vi "Continuous Distillation.vi"() -> ()   [LabVIEW 2017]
uses:
  Halt ContD.vi
  <vilib>/addons/control/pid/pid.llb/PID Advanced (DBL).vi
  <vilib>/addons/control/pid/NI_PID_pid.lvlib
panel:
  out "Condenser Pressure":dbl caption="mbar" format="%#.0f"
  out "Feed Tank Weight":dbl caption="Kg" format="%#.2f"
  in  "Bottoms Flowrate":dbl caption="%"
  in  "Td (Feed Temp)":dbl caption="(min)" format="%.2g"
  in  "Ti (Feed Temp)":dbl=7.0 caption="(min)" format="%.2g"
  in  "Kc (Feed Temp)":dbl=2.0 format="%.2g"
  in  "Reflux Flowrate":dbl caption="ml/min" format="%.1g"
  in  "Feed Flowrate":dbl caption="ml/min" format="%.1g"
  in  "Main Power":bool
  in  "Set Manual Feed Preheater Output":dbl(slide) scale=0.0..100.0
  in  "Manual Control Override":bool
  out "Feed Preheater Output":dbl(slide)=17.346938775510203 scale=0.0..100.0
  in  "Feed Temperature Setpoint":dbl caption="C" format="%.1f"
  out "Feed Temperature":dbl format="%.1g"
  in  "Reboiler Duty":dbl caption="watts"
  out "Tray 11 Temperature":dbl format="%.1g"
  out "Reboiler Temperature":dbl format="%.1g"
  out "Reflux Temperature":dbl format="%.1g"
  out "Overhead Vapor Temperature":dbl caption="C" format="%.1f"
  out "Tray 4 Temperature":dbl caption="C" format="%.1f"
  out "Reboiler Pressure":dbl caption="mbar"
  out "Approximate Bottoms Composition":dbl caption="Wt% CH3OH" format="%.1f"
  out "Approximate Distillate Composition":dbl caption="Wt% CH3OH" format="%.1f"
  in  "stop":bool
  out "Data Point Count":i32
  in  "Specify Time between Data Points (sec)":dbl=1.0
  in  "Cancel Data Collection":bool
  in  "Specify number of data points":i16=1
  in  "Enable 3":bool
  out "Saving Data 3":bool
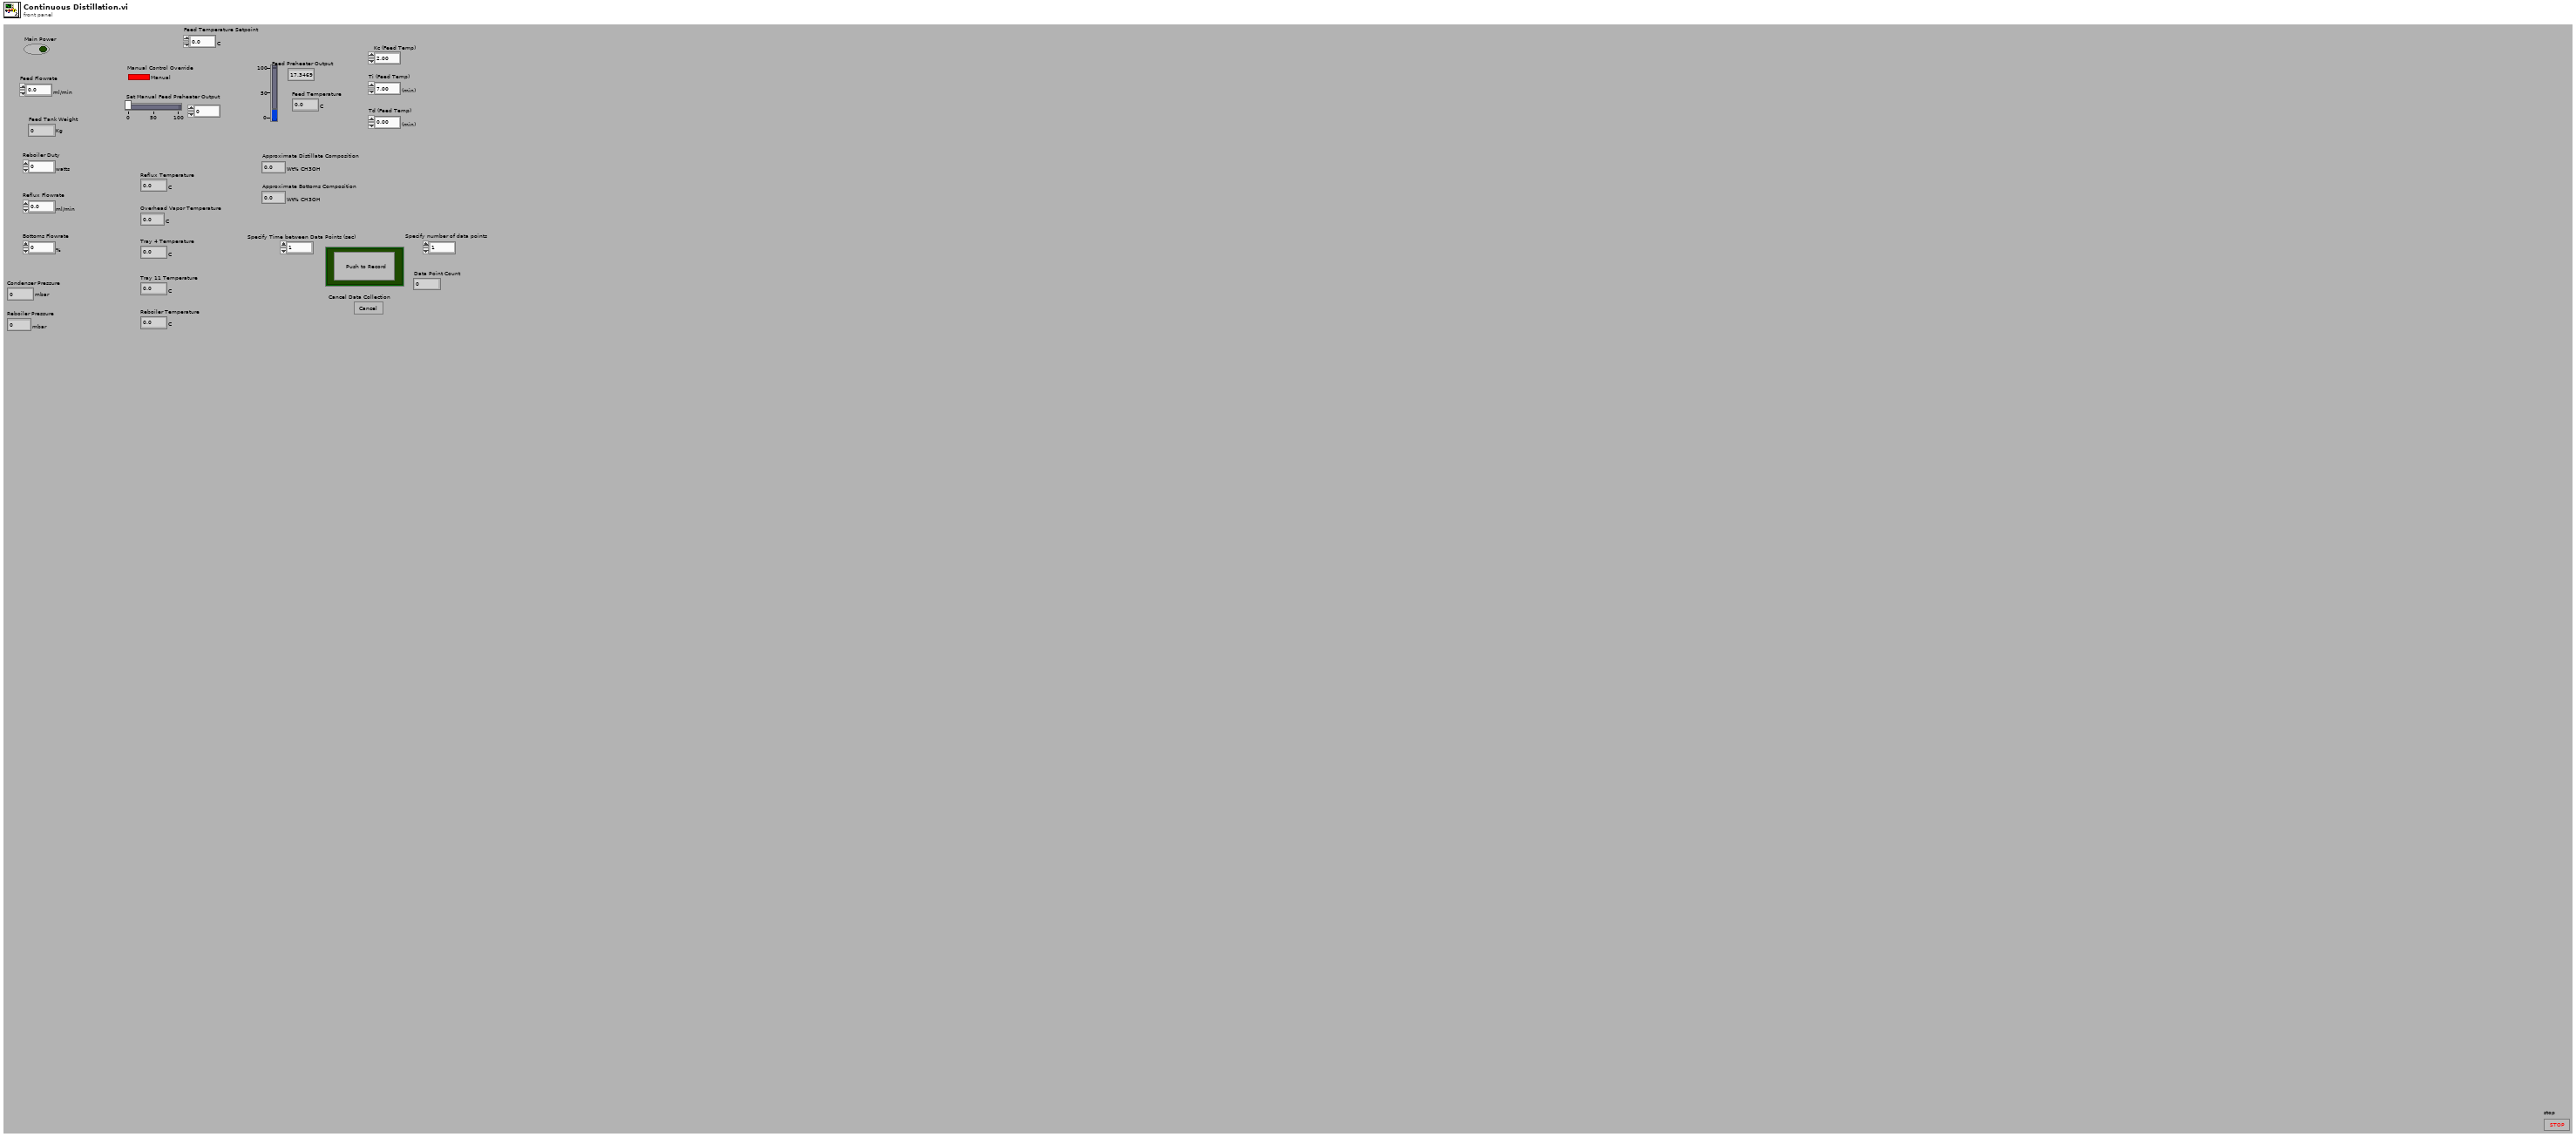
[diagram p1: front panel]
types:
  T1 = cluster{"Kc (Feed Temp)":dbl, "Ti (Feed Temp)":dbl, "Td (Feed Temp)":dbl}
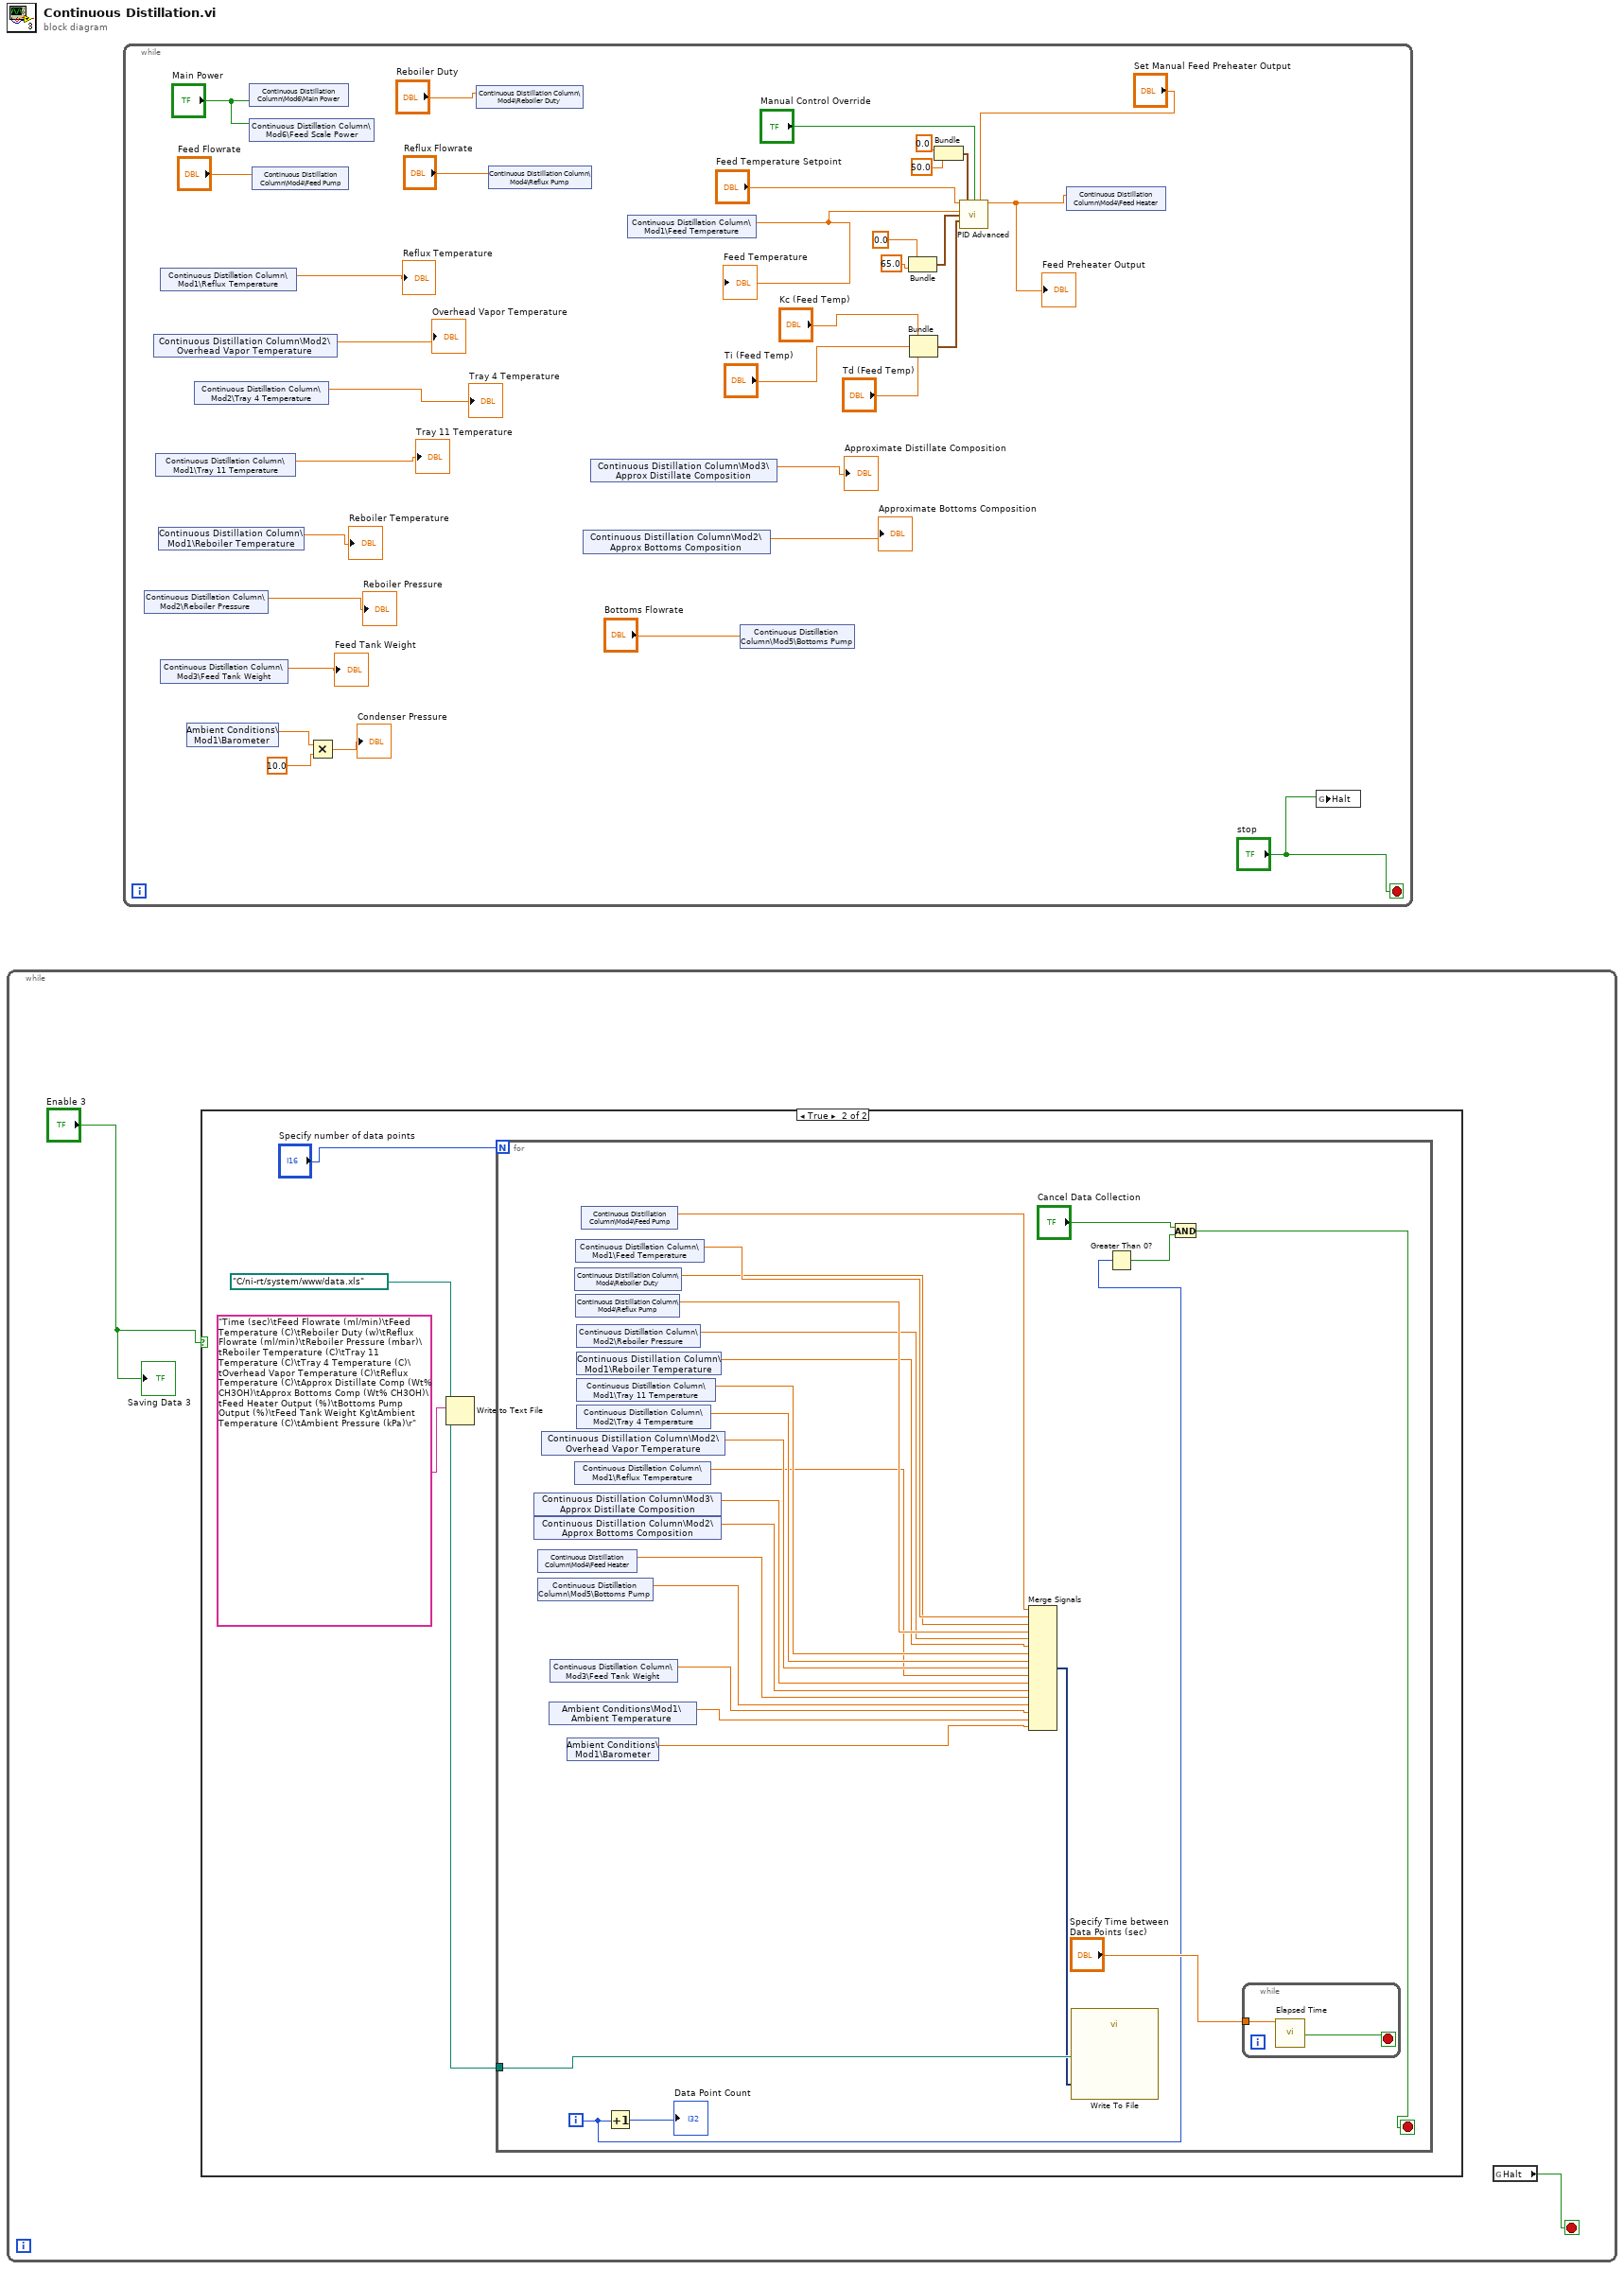
[diagram p0: block diagram]
diagram:
  n1 = while {
    stop <- w1 stop-if-true
    n2 = case shown="True" "Enable 3" {
      frame False {
      }
      frame True {
        w4 = path "C:/ni-rt/system/www/data.xls" ("Filename")
        n3 = Write to Text File(file (use dialog)=w4, text="Time (sec)\tFeed Flowrate (ml/min)\tFeed Temperature (C)\tReboiler Duty (w)\tReflux Flowrate (ml/min)\tReboiler Pressure (mbar)\tReboiler Temperature (C)\tTray 11 Temperature (C)\tTray 4 Temperature (C)\tOverhead Vapor Temperature (C)\tReflux Temperature (C)\tApprox Distillate Comp (Wt% CH3OH)\tApprox Bottoms Comp (Wt% CH3OH)\tFeed Heater Output (%)\tBottoms Pump Output (%)\tFeed Tank Weight Kg\tAmbient Temperature (C)\tAmbient Pressure (kPa)\r") -> ()  [unwired: 2 in, 3 out]
        n4 = for {
          N: "Specify number of data points" -> [_]
          tunnel: w4 -> [w30]
          i -> [w24]
          stop <- w21 stop-if-true
          n5 = shared-variable "Continuous Distillation Column\\Mod3\\Approx Distillate Composition"() -> (w12:dbl)  [unwired: 1 in, 1 out]
          n6 = shared-variable "Continuous Distillation Column\\Mod2\\Approx Bottoms Composition"() -> (w11:dbl)  [unwired: 1 in, 1 out]
          n7 = shared-variable "Continuous Distillation Column\\Mod4\\Feed Heater"() -> (w10:dbl)  [unwired: 1 in, 1 out]
          n8 = shared-variable "Continuous Distillation Column\\Mod5\\Bottoms Pump"() -> (w9:dbl)  [unwired: 1 in, 1 out]
          n9 = shared-variable "Continuous Distillation Column\\Mod2\\Overhead Vapor Temperature"() -> (w18:dbl)  [unwired: 1 in, 1 out]
          n10 = shared-variable "Ambient Conditions\\Mod1\\Ambient Temperature"() -> (w7:dbl)  [unwired: 1 in, 1 out]
          n11 = shared-variable "Continuous Distillation Column\\Mod3\\Feed Tank Weight"() -> (w8:dbl)  [unwired: 1 in, 1 out]
          n12 = shared-variable "Ambient Conditions\\Mod1\\Barometer"() -> (w6:dbl)  [unwired: 1 in, 1 out]
          n13 = shared-variable "Continuous Distillation Column\\Mod4\\Reboiler Duty"() -> (w27:dbl)  [unwired: 1 in, 1 out]
          n14 = shared-variable "Continuous Distillation Column\\Mod1\\Reflux Temperature"() -> (w13:dbl)  [unwired: 1 in, 1 out]
          n15 = shared-variable "Continuous Distillation Column\\Mod1\\Feed Temperature"() -> (w28:dbl)  [unwired: 1 in, 1 out]
          n16 = shared-variable "Continuous Distillation Column\\Mod4\\Reflux Pump"() -> (w20:dbl)  [unwired: 1 in, 1 out]
          n17 = shared-variable "Continuous Distillation Column\\Mod2\\Reboiler Pressure"() -> (w17:dbl)  [unwired: 1 in, 1 out]
          n18 = shared-variable "Continuous Distillation Column\\Mod1\\Reboiler Temperature"() -> (w16:dbl)  [unwired: 1 in, 1 out]
          n19 = shared-variable "Continuous Distillation Column\\Mod1\\Tray 11 Temperature"() -> (w15:dbl)  [unwired: 1 in, 1 out]
          n20 = shared-variable "Continuous Distillation Column\\Mod2\\Tray 4 Temperature"() -> (w14:dbl)  [unwired: 1 in, 1 out]
          n21 = shared-variable "Continuous Distillation Column\\Mod4\\Feed Pump"() -> (w19:dbl)  [unwired: 1 in, 1 out]
          n22 = Increment(x=w24) -> (x+1=→"Data Point Count":i32)
          n23 = Merge Signals(w19, w28, w27, w20, w17, w16, w15, w14, w18, w13, w12, w11, w10, w9, w8, w7, w6) -> (w26:dynamicdata)
          n24 = call "Write To File"("Signals"=w26, "Filename"=w30) -> ()  [unwired: 15 in, 3 out]
          n25 = Greater Than 0?(x=w24) -> (x > 0?=w22:bool)
          n26 = And(x="Cancel Data Collection", y=w22) -> (x .and. y?=w21:bool)
          n27 = while {
            tunnel: "Specify Time between Data Points (sec)" -> [w31]
            stop <- w32 stop-if-true
            n28 = call "Elapsed Time"("Time Target (s)"=w31) -> ("Time has Elapsed"=w32:bool)  [unwired: 11 in, 7 out]
          }
        }
      }
    }
    n29 = global read "Halt ContD.vi" "Halt"() -> (w1:bool)
    "Saving Data 3" <- "Enable 3"
  }
  n30 = while {
    stop <- "stop" stop-if-true
    n31 = shared-variable "Continuous Distillation Column\\Mod2\\Reboiler Pressure"() -> (→"Reboiler Pressure":dbl)  [unwired: 1 in, 1 out]
    n32 = shared-variable "Continuous Distillation Column\\Mod2\\Overhead Vapor Temperature"() -> (→"Overhead Vapor Temperature":dbl)  [unwired: 1 in, 1 out]
    n33 = shared-variable "Continuous Distillation Column\\Mod1\\Tray 11 Temperature"() -> (→"Tray 11 Temperature":dbl)  [unwired: 1 in, 1 out]
    n34 = shared-variable "Continuous Distillation Column\\Mod1\\Reboiler Temperature"() -> (→"Reboiler Temperature":dbl)  [unwired: 1 in, 1 out]
    n35 = shared-variable "Continuous Distillation Column\\Mod1\\Reflux Temperature"() -> (→"Reflux Temperature":dbl)  [unwired: 1 in, 1 out]
    n36 = shared-variable "Continuous Distillation Column\\Mod3\\Feed Tank Weight"() -> (→"Feed Tank Weight":dbl)  [unwired: 1 in, 1 out]
    n37 = shared-variable "Ambient Conditions\\Mod1\\Barometer"() -> (w35:dbl)  [unwired: 1 in, 1 out]
    n38 = shared-variable "Continuous Distillation Column\\Mod2\\Tray 4 Temperature"() -> (→"Tray 4 Temperature":dbl)  [unwired: 1 in, 1 out]
    n39 = shared-variable "Continuous Distillation Column\\Mod6\\Main Power"("Main Power") -> ()  [unwired: 1 in, 1 out]
    n40 = shared-variable "Continuous Distillation Column\\Mod6\\Feed Scale Power"("Main Power") -> ()  [unwired: 1 in, 1 out]
    n41 = shared-variable "Continuous Distillation Column\\Mod4\\Feed Pump"("Feed Flowrate") -> ()  [unwired: 1 in, 1 out]
    n42 = Multiply(x=w35, y=10.0) -> (x*y=→"Condenser Pressure":dbl)
    n43 = shared-variable "Continuous Distillation Column\\Mod4\\Reboiler Duty"("Reboiler Duty") -> ()  [unwired: 1 in, 1 out]
    n44 = shared-variable "Continuous Distillation Column\\Mod4\\Reflux Pump"("Reflux Flowrate") -> ()  [unwired: 1 in, 1 out]
    n45 = shared-variable "Continuous Distillation Column\\Mod2\\Approx Bottoms Composition"() -> (→"Approximate Bottoms Composition":dbl)  [unwired: 1 in, 1 out]
    n46 = shared-variable "Continuous Distillation Column\\Mod3\\Approx Distillate Composition"() -> (→"Approximate Distillate Composition":dbl)  [unwired: 1 in, 1 out]
    n47 = shared-variable "Continuous Distillation Column\\Mod1\\Feed Temperature"() -> (w48:dbl)  [unwired: 1 in, 1 out]
    "Feed Temperature" <- w48
    n48 = shared-variable "Continuous Distillation Column\\Mod5\\Bottoms Pump"("Bottoms Flowrate") -> ()  [unwired: 1 in, 1 out]
    n49 = Bundle(0.0, 65.0) -> (w39:cluster{dbl, dbl})  [unwired: 1 in]
    n50 = Bundle("Kc (Feed Temp)"="Kc (Feed Temp)", "Ti (Feed Temp)"="Ti (Feed Temp)", "Td (Feed Temp)"="Td (Feed Temp)") -> (w56:T1)  [unwired: 1 in]
    n51 = Bundle(0.0, 50.0) -> (w42:cluster{dbl, dbl})  [unwired: 1 in]
    n52 = call-poly <vilib>:"PID Advanced.vi"("setpoint"="Feed Temperature Setpoint", "output range"=w42, "auto? (T)"="Manual Control Override", "manual control"="Set Manual Feed Preheater Output", "process variable"=w48, "setpoint range"=w39, "PID gains"=w56) -> ("output"=w52:dbl)  [unwired: 7 in, 1 out]
    "Feed Preheater Output" <- w52
    n53 = shared-variable "Continuous Distillation Column\\Mod4\\Feed Heater"(w52) -> ()  [unwired: 1 in, 1 out]
    n54 = global write "Halt ContD.vi" "Halt"("stop") -> ()
  }
